vi "DO FGV.vi"(7 "Enum":enum16{"Read", "Write", "Start time", "init"}(ring), 9 "Start Time":timestamp, 10 "DO Channel Names":string[](array[string]), 11 "DO in":bool[](array[boolean])) -> (1 "DO Waveform":waveform(dbl)[](array[waveform]), 2 "DO Channel Names 2":string[](array[string]), 3 "DO out":bool[](array[boolean]))   [LabVIEW 2022 SP3]
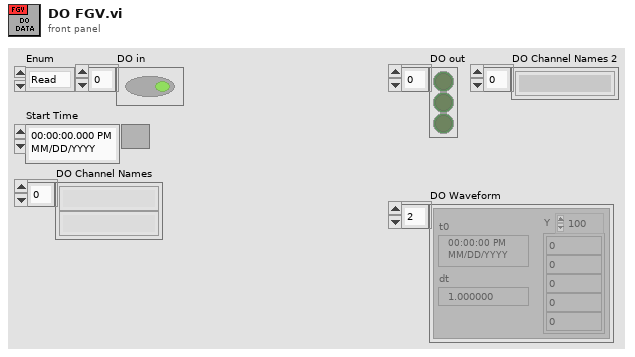
[diagram p1: front panel]
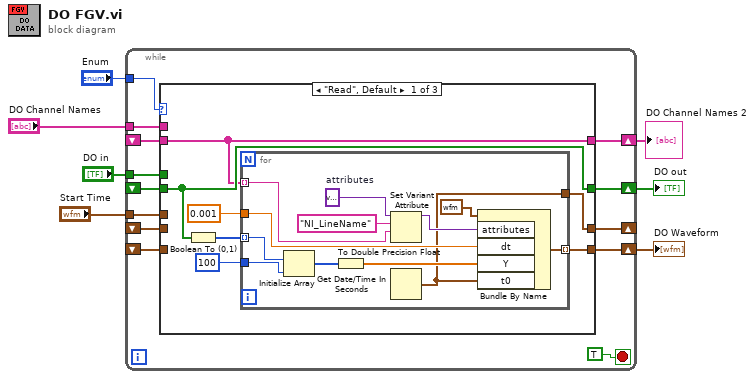
[diagram p0: block diagram]
diagram:
  n1 = while {
    tunnel: "Enum" -> [w19]
    tunnel: "DO in" -> [w18]
    shift-right: [w17] -> w3
    shift-left: _ -> [w16]
    tunnel: "Start Time" -> [w15]
    shift-right: [w14] -> _
    shift-left: _ -> [w13]
    shift-right: [w12] -> w4
    shift-left: _ -> [w11]
    shift-right: [w9] -> w1
    shift-left: _ -> [w10]
    tunnel: "DO Channel Names" -> [w8]
    stop <- TRUE stop-if-true
    n2 = case shown="\"Read\", Default" w19 {
      tunnel: w18 -> [_ w43 _]
      tunnel: [w24 w43 w45] -> w17
      tunnel: w16 -> [w24 _ w45]
      tunnel: w15 -> [_ _ w47]
      tunnel: [w21 w42 w47] -> w14
      tunnel: w13 -> [_ w42 _]
      tunnel: [w23 w41 w46] -> w12
      tunnel: w11 -> [_ w41 w46]
      tunnel: w10 -> [w22 w40 _]
      tunnel: [w22 w40 w44] -> w9
      tunnel: w8 -> [_ _ w44]
      frame "Read", Default {
        n3 = Boolean To (0,1)(Boolean=w24) -> (0, 1=w26:i16[])
        n4 = for {
          tunnel: w26 -> [w38] mode=indexing
          tunnel: [w39] -> w23 mode=indexing
          tunnel: 100 ("Size") -> [w35]
          tunnel: w22 -> [w33] mode=indexing
          tunnel: 0.001 ("dt(sec)") -> [w30]
          tunnel: [w28] -> w21
          w34 = variant  # attributes
          n5 = Initialize Array(w38, w35) -> (w37:i16[])
          n6 = To Double Precision Float(number=w37) -> (double precision float=w36:dbl[])
          n7 = Set Variant Attribute(Variant=w34, name="NI_LineName", value=w33) -> (Variant out=w29:variant)  [unwired: 1 in, 2 out]
          n8 = Get Date/Time In Seconds() -> (seconds since 1Jan1904=w28:timestamp)
          n9 = Bundle By Name(cluster=waveform(dbl) {"t0"=timestamp(0 s since 1904-01-01), "dt"=1.0, "Y"=[]} ("waveform"), "attributes"=w29, "dt"=w30, "Y"=w36, "t0"=w28) -> (w39:waveform(dbl))
        }
      }
      frame "Write" {
      }
      frame "Start time" {
      }
    }
  }
  "DO Waveform" <- w4
  "DO out" <- w3
  "DO Channel Names 2" <- w1
